vi "sub_lane-point_interpolation.vi"(7 "cmd":enum16{"init", "read", "write"}(ring)) -> (0 "graph data":T1(array[cluster]), 1 "error":cluster{"residue-l":dbl, "residue-r":dbl}, 2 "intercept out":cluster{"intercept-l":dbl, "intercept-r":dbl}, 3 "slope out":cluster{"slope-l":dbl, "slope-r":dbl})   [LabVIEW 2019]
uses:
  Ctrl/clamp-result_cmd.ctl
  <vilib>/Analysis/NI_AALPro.lvlib
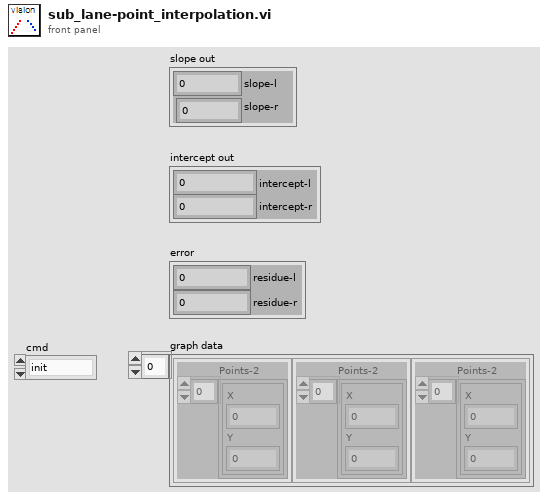
[diagram p1: front panel]
types:
  T1 = cluster{"Points-2":cluster{"X":sgl, "Y":sgl}[]}[]
  T2 = typedef "clamp-result_cmd.ctl" = enum16{"write_clamp_overlay-result", "write_center-distance", "write_clamp_result", "write_threshold_result", "read"}
  T3 = typedef "ROI Descriptor" = cluster{"Global Rectangle":i32[], "Contours":cluster{"ID":enum32{"External", "Internal"}, "Type":u32, "Coordinates":i32[]}[]}
  T4 = cluster{"Edge Coordinates":cluster{"X":sgl, "Y":sgl}[], "dir-data":cluster{"Distance":sgl, "weight-dir":dbl}, "clamp_result":cluster{"Points-1":cluster{"X":sgl, "Y":sgl}[], "Points-2":cluster{"X":sgl, "Y":sgl}[], "Points-3":cluster{cluster{"X":sgl, "Y":sgl}, cluster{"X":sgl, "Y":sgl}}[], "Perpendicular Lines":cluster{cluster{"X":sgl, "Y":sgl}, cluster{"X":sgl, "Y":sgl}}[], "ROI Descriptor out":T3}}
  T5 = cluster{"x-center":dbl, "Image Size":cluster{"x":i32, "y":i32}, "Angle deg":sgl, "Threshold Range":cluster{"Lower value":sgl, "Upper value":sgl}}
  T6 = cluster{"Points-1":cluster{"X":sgl, "Y":sgl}[], "Points-2":cluster{"X":sgl, "Y":sgl}[], "Points-3":cluster{cluster{"X":sgl, "Y":sgl}, cluster{"X":sgl, "Y":sgl}}[], "Perpendicular Lines":cluster{cluster{"X":sgl, "Y":sgl}, cluster{"X":sgl, "Y":sgl}}[], "ROI Descriptor out":T3}
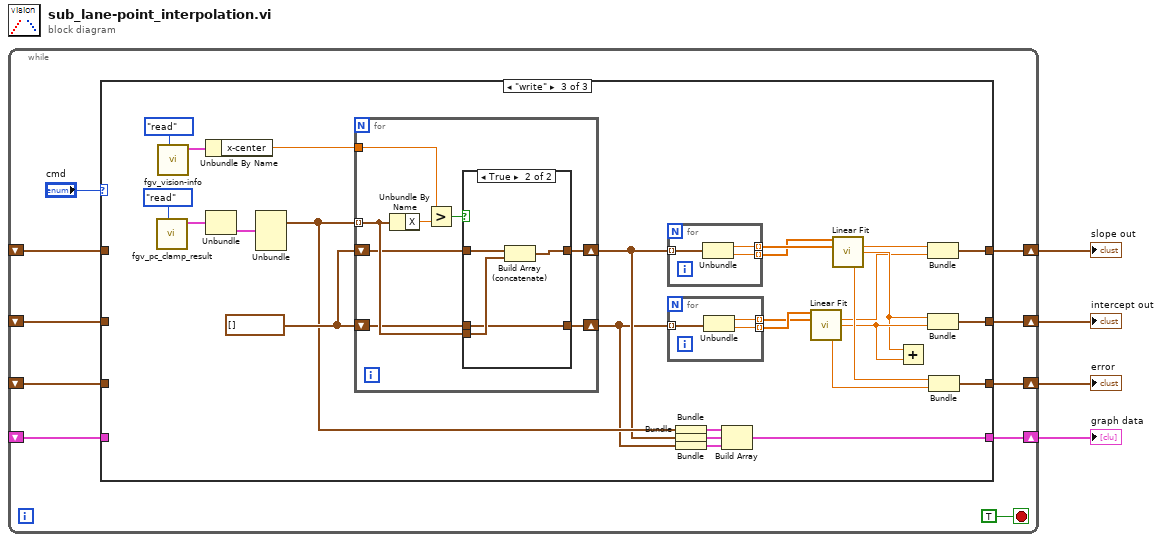
[diagram p0: block diagram]
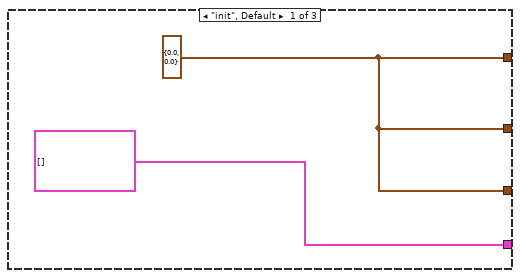
[diagram p2: hidden frame]
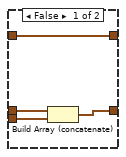
[diagram p4: hidden frame]
diagram:
  n1 = while {
    shift-right: [w12] -> w4
    shift-left: _ -> [w9]
    shift-right: [w11] -> w3
    shift-left: _ -> [w8]
    shift-right: [w10] -> w2
    shift-left: _ -> [w7]
    shift-right: [w6] -> w1
    shift-left: _ -> [w5]
    stop <- TRUE stop-if-true
    n2 = case shown="\"write\"" "cmd" {
      tunnel: [w16 w20 w24] -> w12
      tunnel: [w16 w19 w23] -> w11
      tunnel: [w16 w18 w22] -> w10
      tunnel: w9 -> [_ w20 _]
      tunnel: w8 -> [_ w19 _]
      tunnel: w7 -> [_ w18 _]
      tunnel: [T1 [] w17 w21] -> w6
      tunnel: w5 -> [_ w17 _]
      frame "init", Default {
        w16 = cluster{"slope":dbl, "slope":dbl} {"slope"=0.0, "slope"=0.0}
      }
      frame "read" {
      }
      frame "write" {
        w35 = cluster{"X":sgl, "Y":sgl}[] []
        n3 = call "fgv_pc_clamp_result.vi"("cmd"=clamp-result_cmd."read") -> ("clamp result out"=w36:T4)  [unwired: 7 in, 3 out]
        n4 = call "fgv_vision-info.vi"("cmd"=enum16{"read", "write"}."read") -> ("image info out"=w33:T5)  [unwired: 10 in]
        n5 = Unbundle By Name(w33) -> ("x-center"=w34:dbl)
        n6 = Unbundle(w36) -> ("clamp_result"=w37:T6)  [unwired: 2 out]
        n7 = Unbundle(w37) -> ("Points-2"=w30:cluster{"X":sgl, "Y":sgl}[])  [unwired: 4 out]
        n8 = for {
          tunnel: w30 -> [w58] mode=indexing
          shift-right: [w56] -> w29
          shift-left: w35 -> [w57]
          shift-right: [w55] -> w28
          shift-left: w35 -> [w54]
          tunnel: w34 -> [w61]
          n9 = Unbundle By Name(w58) -> ("X"=w60:sgl)
          n10 = Greater?(x=w61, y=w60) -> (0:w59:bool)
          n11 = case shown="True" w59 {
            tunnel: w58 -> [w62 w67]
            tunnel: w57 -> [w65 w69]
            tunnel: [w65 w68] -> w56
            tunnel: [w64 w66] -> w55
            tunnel: w54 -> [w63 w66]
            frame False {
              n12 = Build Array (concatenate)(w63, w62) -> (w64:cluster{"X":sgl, "Y":sgl}[])
            }
            frame True {
              n13 = Build Array (concatenate)(w69, w67) -> (w68:cluster{"X":sgl, "Y":sgl}[])
            }
          }
        }
        n14 = for {
          tunnel: w29 -> [w53] mode=indexing
          tunnel: [w52] -> w38 mode=indexing
          tunnel: [w51] -> w39 mode=indexing
          n15 = Unbundle(w53) -> ("X"=w51:sgl, "Y"=w52:sgl)
        }
        n16 = for {
          tunnel: w28 -> [w50] mode=indexing
          tunnel: [w49] -> w41 mode=indexing
          tunnel: [w48] -> w40 mode=indexing
          n17 = Unbundle(w50) -> ("X"=w48:sgl, "Y"=w49:sgl)
        }
        n18 = Bundle("Points-2"=w30) -> (w25:cluster{"Points-2":cluster{"X":sgl, "Y":sgl}[]})  [unwired: 1 in]
        n19 = Bundle(w29) -> (w26:cluster{cluster{"X":sgl, "Y":sgl}[]})  [unwired: 1 in]
        n20 = Bundle(w28) -> (w27:cluster{cluster{"X":sgl, "Y":sgl}[]})  [unwired: 1 in]
        n21 = Build Array(w25, w26, w27) -> (w21:T1)
        n22 = call <vilib>:"Linear Fit.vi"("Y"=w41, "X"=w40) -> ("slope"=w43:dbl, "intercept"=w45:dbl, "residue"=w47:dbl)  [unwired: 9 in, 2 out]
        n23 = call <vilib>:"Linear Fit.vi"("Y"=w38, "X"=w39) -> ("slope"=w42:dbl, "intercept"=w44:dbl, "residue"=w46:dbl)  [unwired: 9 in, 2 out]
        n24 = Add(x=w44, y=w45) -> ()  [unwired: 1 out]
        n25 = Bundle("slope"=w42, "slope"=w43) -> (w24:cluster{"slope":dbl, "slope":dbl})  [unwired: 1 in]
        n26 = Bundle("intercept"=w44, "intercept"=w45) -> (w23:cluster{"intercept":dbl, "intercept":dbl})  [unwired: 1 in]
        n27 = Bundle("residue"=w46, "residue"=w47) -> (w22:cluster{"residue":dbl, "residue":dbl})  [unwired: 1 in]
      }
    }
  }
  "slope out" <- w4
  "intercept out" <- w3
  "error" <- w2
  "graph data" <- w1
